vi "Create Frame Pattern Script.vi"(8 "error in (no error)":errorcluster, 10 "SPI_FRM_Config":T1 {"Addr" format="%x"; "Data" format="%x"}, 11 "SPI_Frame_Read_Data in":refnum<class "SPI_Frame_Read_Data.lvclass">) -> (0 "error out":errorcluster, 3 "SPI_Frame_Read_Data out":refnum<class "SPI_Frame_Read_Data.lvclass">)   [LabVIEW 2018, in "SPI_Frame_Read_Data.lvclass"]
uses:
  SPI_Frame_Read_Data.lvclass
  C:/P4 Workspace/PC Client/Solutions/5g_eap/HiSi/trunk/1.0/BML_Pattern_Gen_Refactor/SPI/SPI Frame Root/SPI_Frame_Root.lvclass
  Config Read SPI/SPI_FRM_Config.ctl
  Classes/Config_Read/RW_Option.ctl
  Config Read SPI/SPI_Mode.ctl
  SPI_Frame_Read_Data.lvclass/SPI_Frame_Read_Data.ctl
  SPI Frame Root/SPI_Frame_Root.lvclass/SPI_Frame_Root.ctl
  Classes/BML_Frame_Root/Special Frame.ctl
  SPI_Frame_Read_Collect/SPI_Frame_Read_Collect.lvclass
  SPI_Frame_Read_Capture/SPI_Frame_Read_Capture.lvclass
  SPI Frame Root/SPI_Frame_Root.lvclass
  Classes/BML_Frame_Root/BML_Frame_Root.lvclass
  Classes/Config_Read/Config_Read_BML.lvclass
  Config Read SPI/Config_Read_SPI.lvclass
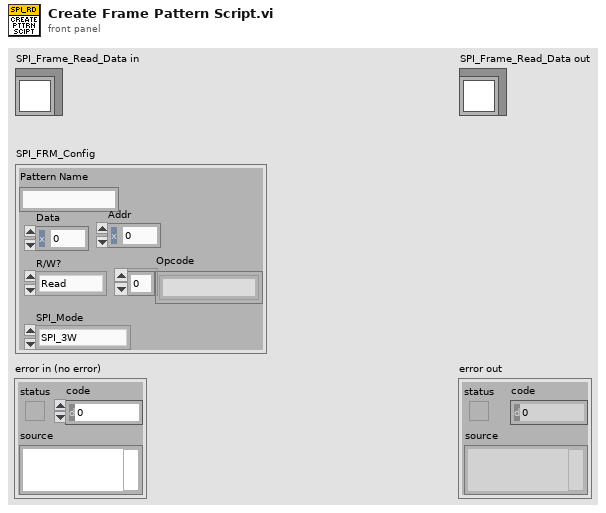
[diagram p1: front panel]
types:
  T1 = typedef "Config_Read_SPI.lvclass/SPI_FRM_Config.ctl" = cluster{"Pattern Name":string, "Data":u16, "Addr":u16, "R/W?":T2, "Opcode":string[], "SPI_Mode":T3}
  T2 = typedef "Config_Read_BML.lvclass/RW_Option.ctl" = enum16{"Read", "Write", "R/W"}
  T3 = typedef "Config_Read_SPI.lvclass/SPI_Mode.ctl" = enum16{"SPI_3W", "SPI_4W"}
  T4 = typedef "BML_Frame_Root.lvclass/Special Frame.ctl" = enum16{"Sync Header", "Protocol Header", "SW Trig", "SetID State", "Out SetID State", "SW Reset", "Wait", "SPI 4W FRM Start", "SPI 4W Wait", "SPI 4W FRM End", "SPI 4W Write Cmd", "SPI RD Collect Cmd", "SPI RD Value Cmd", "SPI 3W FRM Start", "SPI 3W Write Cmd", "SPI 3W FRM End", "SPI 3W Wait", "SPI 3W RD Cmd"}
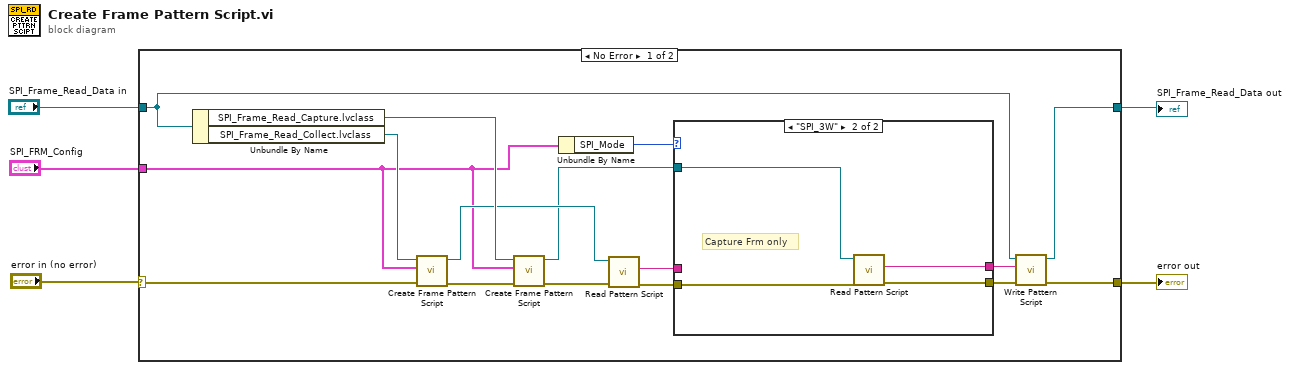
[diagram p0: block diagram]
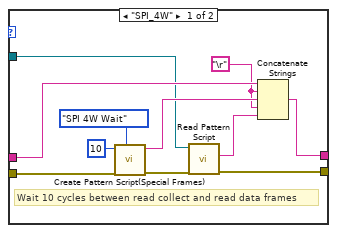
[diagram p2: hidden frame]
diagram:
  n1 = case shown="No Error" "error in (no error)" {
    selector: "error in (no error)" -> [w11 w38]
    tunnel: "SPI_Frame_Read_Data in" -> [w14 w37]
    tunnel: [w15 w38] -> w1
    tunnel: [w13 w37] -> w2
    tunnel: "SPI_FRM_Config" -> [w7 _]
    frame No Error {
      n2 = Unbundle By Name(w14) -> ("SPI_Frame_Read_Capture.lvclass"=w17:refnum<class "SPI_Frame_Read_Capture.lvclass">, "SPI_Frame_Read_Collect.lvclass"=w20:refnum<class "SPI_Frame_Read_Collect.lvclass">)
      n3 = call-dynamic "Create Frame Pattern Script.vi"("error in (no error)"=w11, "SPI_FRM_Config"=w7, "SPI_Frame_Read_Collect in"=w20) -> ("error out"=w21:errorcluster, "SPI_Frame_Read_Collect out"=w9:refnum<class "SPI_Frame_Read_Collect.lvclass">)  [unwired: 7 in]
      n4 = call-dynamic "Create Frame Pattern Script.vi"("error in (no error)"=w21, "SPI_FRM_Config"=w7, "SPI_Frame_Read_Capture in"=w17) -> ("error out"=w10:errorcluster, "SPI_Frame_Read_Capture out"=w8:refnum<class "SPI_Frame_Read_Capture.lvclass">)  [unwired: 7 in]
      n5 = Unbundle By Name(w7) -> ("SPI_Mode"=w6:T3)
      n6 = call "Read Pattern Script.vi"("error in (no error)"=w10, "SPI_Frame_Root in"=w9) -> ("error out"=w19:errorcluster, "Pattern Script"=w18:string)  [unwired: 7 in, 1 out]
      n7 = case shown="\"SPI_3W\"" w6 {
        tunnel: w19 -> [w31 w33]
        tunnel: w18 -> [w29 _]
        tunnel: [w25 w36] -> w16
        tunnel: [w24 w34] -> w12
        tunnel: w8 -> [w23 w35]
        frame "SPI_4W" {
          w27 = "\r"
          # "Wait 10 cycles between read collect and read data frames"
          n8 = call "Create Pattern Script(Special Frames).vi"("Special Frame Type"=Special_Frame."SPI 4W Wait", "error in (no error)"=w31, "Num of Timeset"=u32 10) -> ("error out"=w32:errorcluster, "string out"=w28:string)  [unwired: 7 in]
          n9 = call "Read Pattern Script.vi"("error in (no error)"=w32, "SPI_Frame_Root in"=w23) -> ("error out"=w25:errorcluster, "Pattern Script"=w26:string)  [unwired: 7 in, 1 out]
          n10 = Concatenate Strings(w29, w27, w28, w27, w26) -> (w24:string)
        }
        frame "SPI_3W" {
          # "Capture Frm only"
          n11 = call "Read Pattern Script.vi"("error in (no error)"=w33, "SPI_Frame_Root in"=w35) -> ("error out"=w36:errorcluster, "Pattern Script"=w34:string)  [unwired: 7 in, 1 out]
        }
      }
      n12 = call "Write Pattern Script.vi"("error in (no error)"=w16, "Pattern Script"=w12, "SPI_Frame_Root in"=w14) -> ("error out"=w15:errorcluster, "SPI_Frame_Root out"=w13:refnum<class "SPI_Frame_Read_Data.lvclass">)  [unwired: 7 in]
    }
    frame Error {
    }
  }
  "error out" <- w1
  "SPI_Frame_Read_Data out" <- w2
